vi "USB9825_AD_UnLink.vi"(8 "Error In":errorcluster caption="错误输入", 11 "hDevice":i32) -> (0 "Error Out":errorcluster caption="错误输出")   [LabVIEW 2015, in "DAQ.lvlib"]
uses:
  DAQ.lvlib
  USB9825.DLL
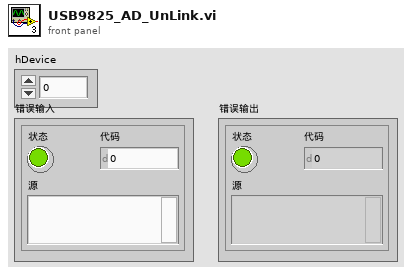
[diagram p1: front panel]
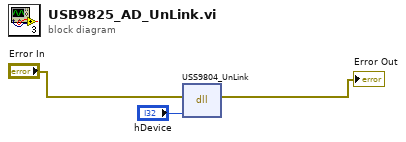
[diagram p0: block diagram]
diagram:
  n1 = dll-call lib="PTH2sabs CYexinrongWorkplace\t普密斯Thickness-measurementBiometry_alpha3 bolihouduSub VIsDAQUSB9825.dll" fn="USS9804_UnLink"(error in="Error In", "hDevice"="hDevice") -> (error out=→"Error Out":errorcluster)  [unwired: 4 in, 1 out]
